vi "Do.vi"(8 "error in (no error)":errorcluster, 10 "Actor in":refnum<class "Actor.lvclass">, 11 "ReadDeviceState Msg":refnum<class "ReadDeviceState Msg.lvclass">) -> (0 "error out":errorcluster, 2 "Actor out":refnum<class "Actor.lvclass">)   [LabVIEW 2019, in "BASE.Device.lvlib" / "ReadDeviceState Msg.lvclass"]
doc: "This VI delivers the message to the actor by calling the appropriate method(s) on the actor."
uses:
  ReadDeviceState Msg.lvclass
  <vilib>/ActorFramework/Actor/Actor.lvclass
  BASE.Device/BASE.Device.lvclass
  D:/Program Files (x86)/National Instruments/LabVIEW 2019/vi.lib/ActorFramework/Actor/Actor.lvclass
  ReadDeviceState Msg.lvclass/ReadDeviceState Msg.ctl
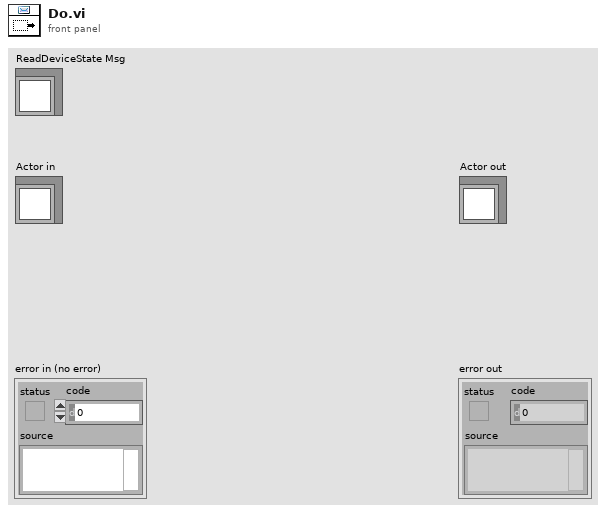
[diagram p1: front panel]
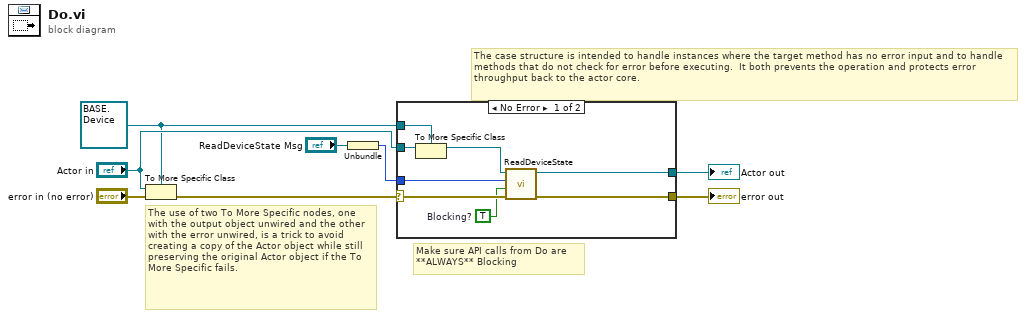
[diagram p0: block diagram]
diagram:
  w2 = refnum<class "BASE.Device.lvclass"> refnum ("Actor in")
  # "Make sure API calls from Do are\n**ALWAYS** Blocking"
  # "The use of two To More Specific nodes, one with the output object unwired and the other with the error unwired, is a trick to avoid creating a copy of the Actor object while still preserving the original Actor object if the To More Specific fails."
  # "The case structure is intended to handle instances where the target method has no error input and to handle methods that do not check for error before executing.  It both prevents the operation and protects error throughput back to the actor core."
  n1 = To More Specific Class(target class=w2, reference="Actor in", error in="error in (no error)") -> (error out=w6:errorcluster)  [unwired: 1 out]
  n2 = Unbundle("ReadDeviceState Msg") -> (w1:i32)
  n3 = case shown="No Error" w6 {
    selector: w6 -> [w14 w18]
    tunnel: [w16 w18] -> w5
    tunnel: [w15 w17] -> w4
    tunnel: "Actor in" -> [w13 w17]
    tunnel: w2 -> [w12 _]
    tunnel: w1 -> [w10 _]
    frame No Error {
      w9 = TRUE  # Blocking?
      n4 = To More Specific Class(target class=w12, reference=w13) -> (specific class reference=w11:refnum<class "BASE.Device.lvclass">)  [unwired: 1 in, 1 out]
      n5 = call "ReadDeviceState.vi"("error in (no error)"=w14, "Blocking?"=w9, "Timeout (5000 ms)"=w10, "BASE.Device in"=w11) -> ("error out"=w16:errorcluster, "BASE.Device out"=w15:refnum<class "BASE.Device.lvclass">)  [unwired: 6 in]
    }
    frame Error {
      # "If type check fails, pass the original object out again."
    }
  }
  "error out" <- w5
  "Actor out" <- w4
